vi "Kalman Filter Altitude.vi"   [LabVIEW 2014, in "Observer Library.lvlib" / "Kalman Filter Altitude.lvclass"]
uses:
  Kalman Filter Altitude.lvclass
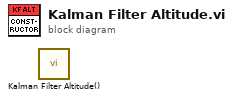
[diagram p0: block diagram]
diagram:
  n1 = call "Kalman Filter Altitude().vi"() -> ()  [unwired: 11 in, 1 out]
